vi "getActiveItems.vi"(11 "Enum in":refnum<vi>) -> (3 "array w/ subset deleted":string[](array[string]))   [LabVIEW 2013]
uses:
  <userlib>/_OpenG.lib/array/array.llb/Delete Elements from 1D Array (String)__ogtk.vi
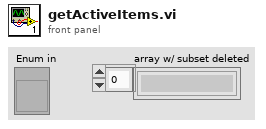
[diagram p1: front panel]
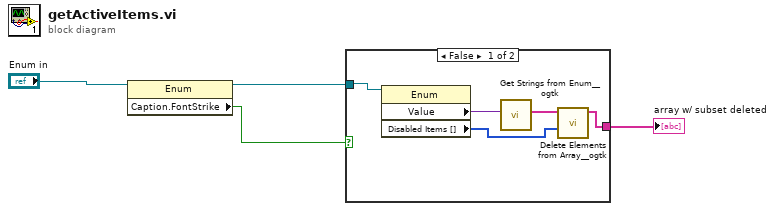
[diagram p0: block diagram]
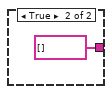
[diagram p2: hidden frame]
diagram:
  n1 = property class="Enum"(reference="Enum in") -> (reference out=w2:refnum<vi>, "Caption.FontStrike"=w3:bool)  [unwired: 1 in, 1 out]
  n2 = case shown="False" w3 {
    tunnel: w2 -> [w9 _]
    tunnel: [w6 string[] [] ("array w/ subset deleted")] -> w4
    frame False {
      n3 = property class="Enum"(reference=w9) -> ("Value"=w5:variant, "Disabled Items []"=w7:i32[])  [unwired: 1 in, 2 out]
      n4 = call <userlib>:"Get Strings from Enum__ogtk.vi"("Enum"=w5) -> ("Enum Strings"=w8:string[])  [unwired: 7 in, 3 out]
      n5 = call-poly <userlib>:"Delete Elements from Array__ogtk.vi"("indices"=w7, "array"=w8) -> ("array w/ subset deleted"=w6:string[])  [unwired: 8 in, 1 out]
    }
    frame True {
    }
  }
  "array w/ subset deleted" <- w4
